vi "Receive Datagram.vi"(8 "error in (no error)":errorcluster, 10 "transfer group id":i32, 11 "UDP Transceiver in":refnum<class "UDP Transceiver.lvclass">) -> (0 "error out":errorcluster, 1 "transfer data":string, 2 "transfer id":i32, 3 "UDP Transceiver out":refnum<class "UDP Transceiver.lvclass">, 4 "valid":bool)   [LabVIEW 2017, in "UDP.lvlib" / "UDP Transceiver.lvclass"]
uses:
  UDP Transceiver.lvclass
  UDP Transceiver.lvclass/UDP Transceiver.ctl
  <vilib>/Utility/error.llb/Clear Errors.vi
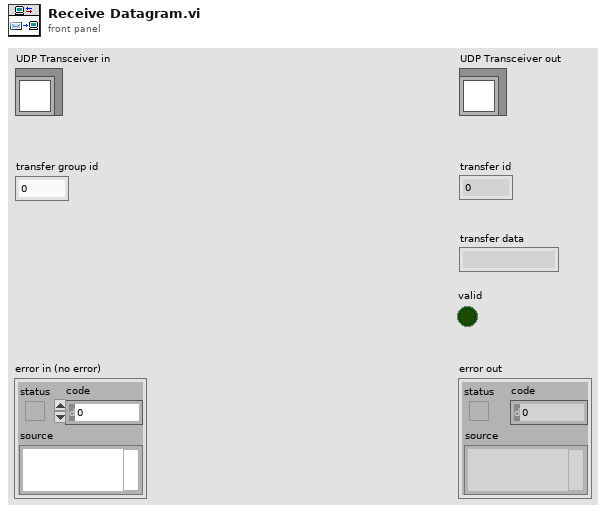
[diagram p1: front panel]
types:
  T1 = typedef "UDP.lvlib/UDP Transceiver.lvclass/Transfer Group Parameters.ctl" = cluster{"transfers":T2[], "max size":i32, "timeout":i32}
  T2 = typedef "UDP.lvlib/UDP Transceiver.lvclass/Transfer Parameters.ctl" = cluster{"group offset":u64, "size":u64, "address":u32, "port":u16}
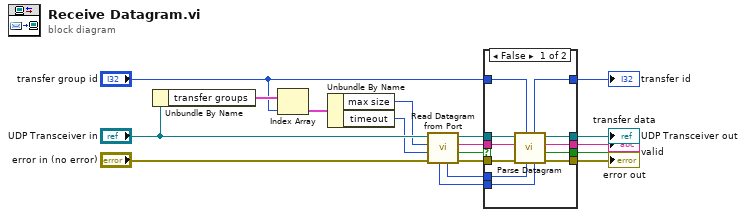
[diagram p0: block diagram]
diagram:
  n1 = Unbundle By Name("UDP Transceiver in") -> ("transfer groups"=w7:T1[])
  n2 = Index Array(array=w7, index="transfer group id") -> (element=w5:T1)
  n3 = Unbundle By Name(w5) -> ("max size"=w2:i32, "timeout"=w1:i32)
  n4 = call "Read Datagram from Port.vi"("error in (no error)"="error in (no error)", "timeout ms (25000)"=w1, "max size (548)"=w2, "UDP Transceiver in"="UDP Transceiver in") -> ("error out"=w16:errorcluster, "timed out?"=w4:bool, "data"=w14:string, "UDP Transceiver out"=w17:refnum<class "UDP Transceiver.lvclass">, "source port"=w13:u16, "source address"=w12:u32)  [unwired: 2 in]
  n5 = case shown="False" w4 {
    tunnel: w17 -> [w29 w30]
    tunnel: w16 -> [w28 w31]
    tunnel: [w27 w30] -> w15
    tunnel: w14 -> [w26 _]
    tunnel: "transfer group id" -> [w25 _]
    tunnel: w13 -> [w24 _]
    tunnel: w12 -> [w23 _]
    tunnel: [w22 _] -> w11
    tunnel: [w21 _] -> w10
    tunnel: [w20 w31] -> w9
    tunnel: [w19 _] -> w8
    frame False {
      n6 = call-dynamic "Parse Datagram.vi"("source address"=w23, "source port"=w24, "transfer group id"=w25, "error in (no error)"=w28, "datagram"=w26, "UDP Transceiver in"=w29) -> ("error out"=w20:errorcluster, "valid"=w21:bool, "transfer data"=w19:string, "UDP Transceiver out"=w27:refnum<class "UDP Transceiver.lvclass">, "transfer id"=w22:i32)  [unwired: 1 in]
    }
    frame True {
    }
  }
  "error out" <- w9
  "UDP Transceiver out" <- w15
  "transfer id" <- w11
  "transfer data" <- w8
  "valid" <- w10
